vi "TrentVisionTest.vi"() -> ()   [LabVIEW 2011]
uses:
  <vilib>/Analysis/1siggen.llb/Ramp Pattern by Samples.vi
  <vilib>/Analysis/NI_AALBase.lvlib
  <vilib>/robotics/Navigation/shared/WorldMap/OccupancyGridWorldMap/NI_Robotics_OccupancyGridWorldMap.lvclass
panel:
  out "Image Out 2":T1(plugin-control)
  out "Lines Calibrated (Shape Detection 1) 2":T2(array[cluster]) {"End Point"."Y" format="%.2f"; "End Point"."X" format="%.2f"; "Start Point"."Y" format="%.2f"; "Start Point"."X" format="%.2f"}
  in  "ALL STOP":bool
  out "Started Scanning":bool
  in  "Step Over":bool
  out "Elapsed Time to Scan for First Time (sec)":dbl
  in  "Step Enable":bool
  out "Occupancy Grid":dbl[][](graph)
  out "XY Graph":cluster{dbl[], dbl[]}[](graph)
  in  "x Offset":i32
  in  "y Offset":i32
  in  "end point (135°)":dbl=100.0
  in  "Resulotion Controller\n1m = 10 units\n30m = 300 units (default)":i32=300
  in  "y start":i32
  in  "x start":i32
  out "Lines Calibrated (Shape Detection 1)":T2(array[cluster]) {"End Point"."Y" format="%.2f"; "End Point"."X" format="%.2f"; "Start Point"."Y" format="%.2f"; "Start Point"."X" format="%.2f"}
  out "Image Out":T1(plugin-control)
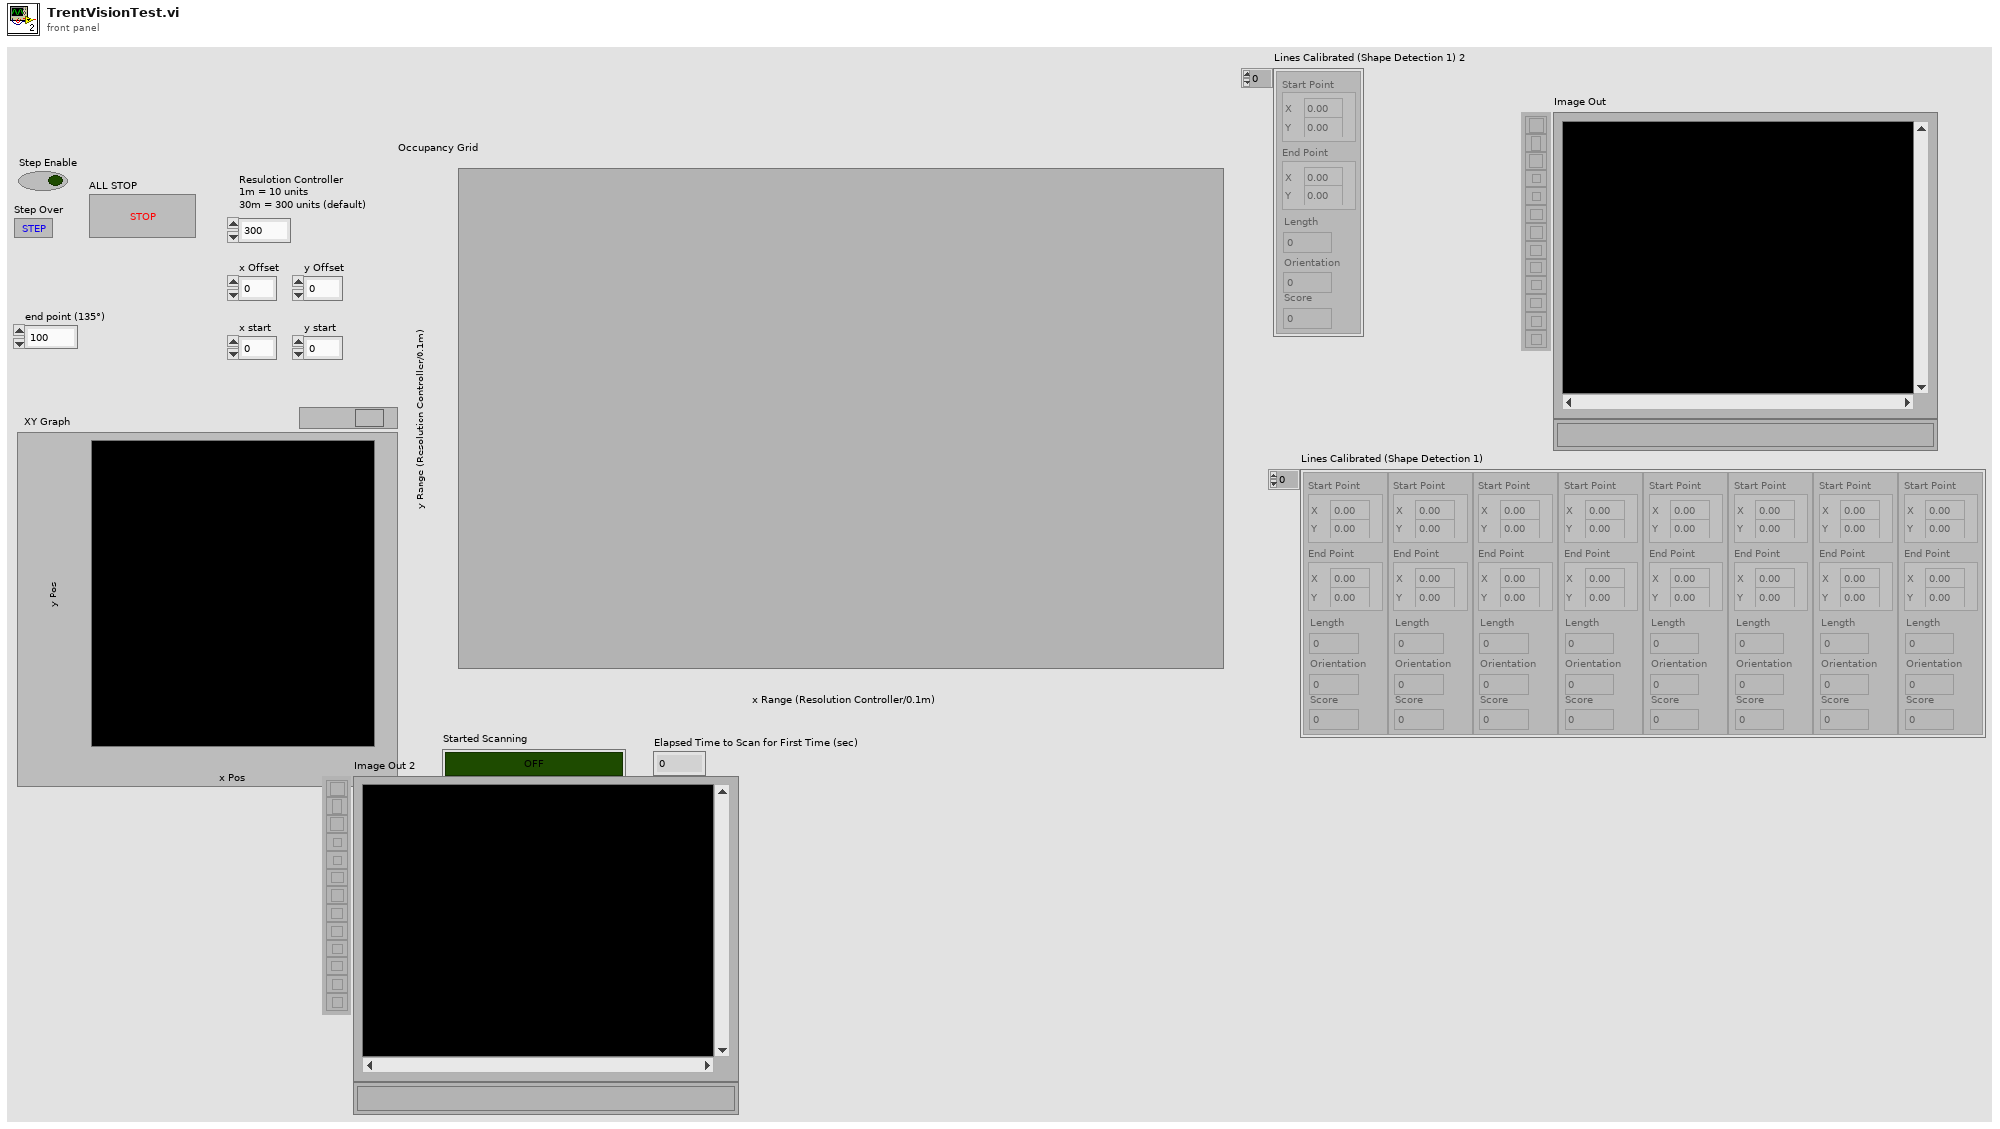
[diagram p1: front panel]
types:
  T1 = typedef "IMAQ Image.ctl" = refnum<image>
  T2 = cluster{"Start Point":cluster{"X":sgl, "Y":sgl}, "End Point":cluster{"X":sgl, "Y":sgl}, "Length":dbl, "Orientation":dbl, "Score":dbl}[]
  T3 = typedef "Image Type" = u32
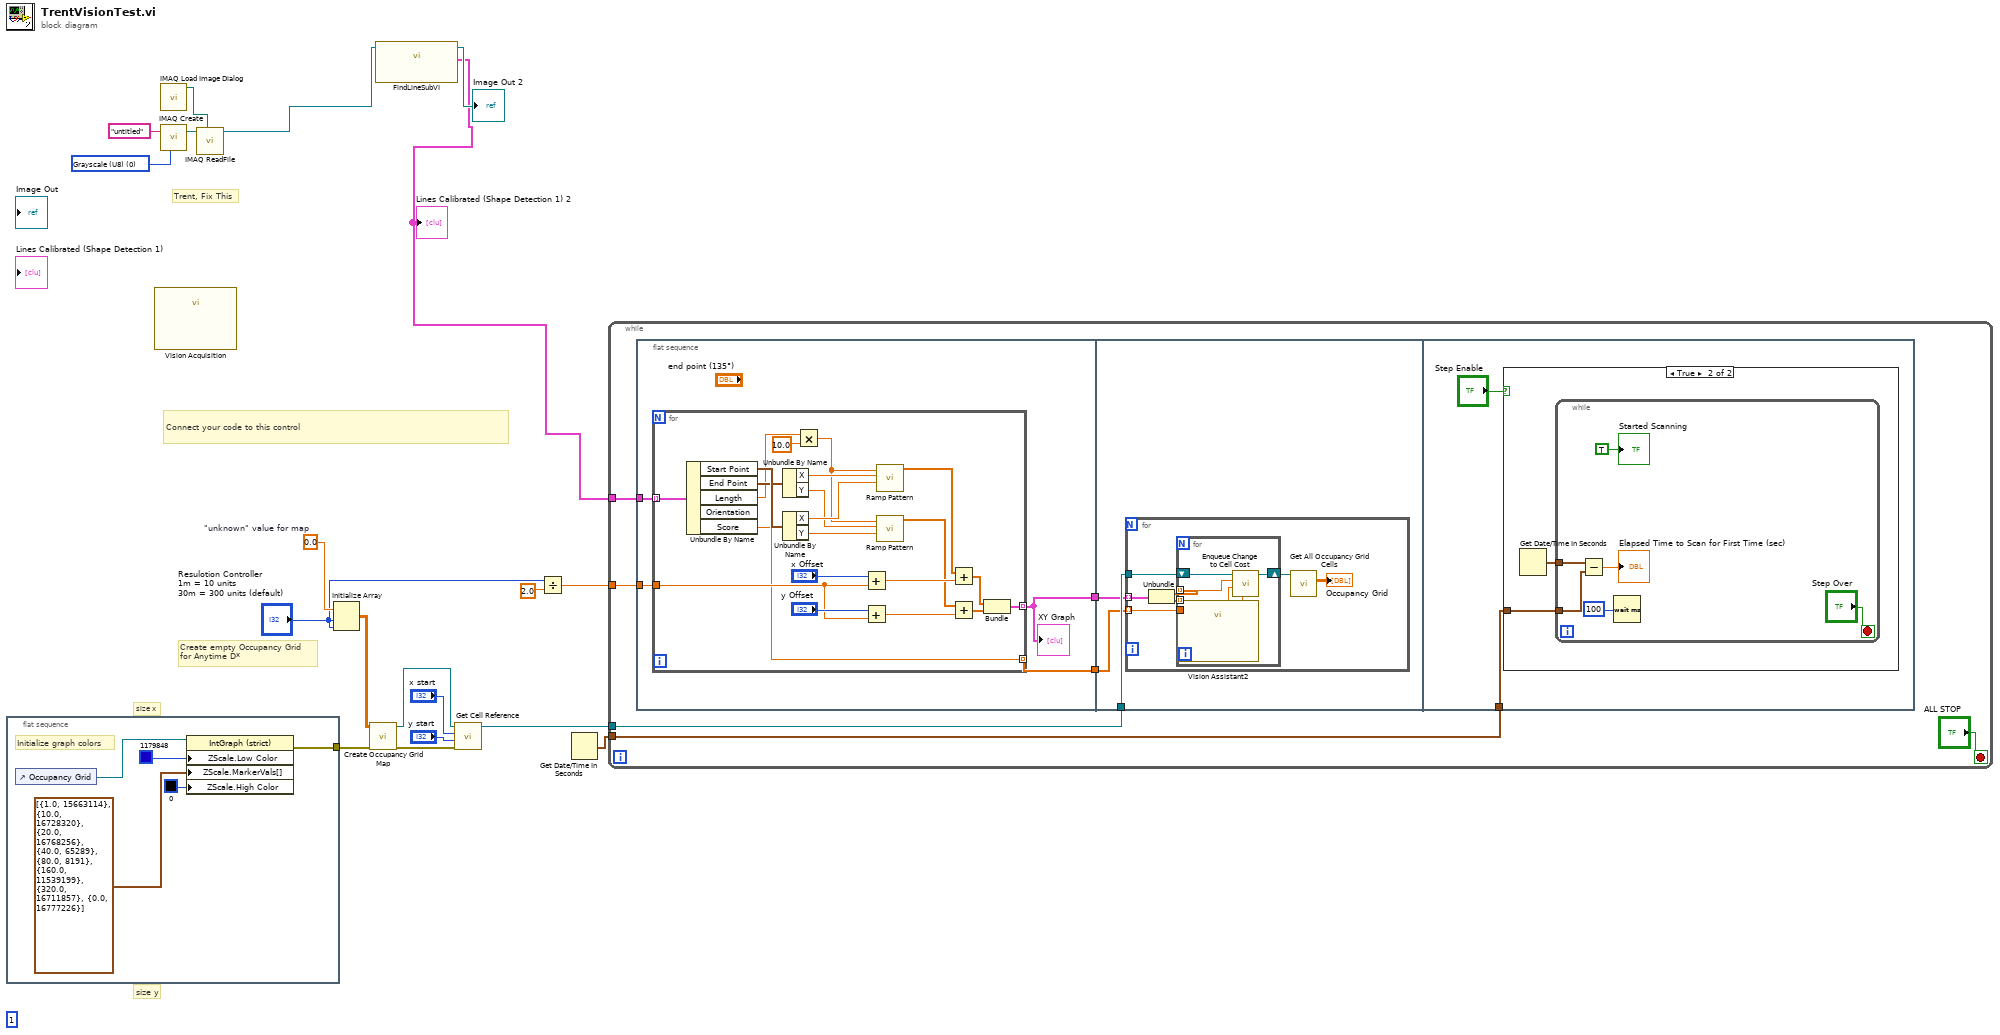
[diagram p0: block diagram]
diagram:
  w4 = T3 0 items=["Grayscale (U8)", "Grayscale (I16)", "Grayscale (SGL)", "Complex (CSG)", "RGB (U32)", "HSL (U32)", "RGB (U64)", "Grayscale (U16)"] ("Image Type")
  (unwired) 1
  w19 = 0.0  # "unknown" value for map
  # "Trent, Fix This"
  # "Connect your code to this control"
  # "size y"
  # "size x"
  # "Create empty Occupancy Grid\nfor Anytime D*"
  n1 = flat-sequence {
    tunnel: [w21] -> w13
    frame #0 {
      # "Initialize graph colors"
      n2 = control-ref of="Occupancy Grid"() -> (w20:refnum<vi>)
      n3 = property on="Property Node" class="IntGraph (strict)"(reference=w20, "ZScale.Low Color"=u32 1179848, "ZScale.MarkerVals[]"=cluster{dbl, u32}[] [{1.0, 15663114}, {10.0, 16728320}, {20.0, 16768256}, {40.0, 65289}, {80.0, 8191}, {160.0, 11539199}, {320.0, 16711857}, {0.0, 16777226}], "ZScale.High Color"=u32 0) -> (error out=w21:errorcluster)  [unwired: 1 in, 1 out]
    }
  }
  n4 = call "Vision Acquisition"() -> ()  [unwired: 20 in]
  n5 = call "IMAQ Load Image Dialog"() -> ("Path"=w5:path)  [unwired: 9 in, 2 out]
  n6 = call "IMAQ Create"("Image Name"="untitled", "Image Type"=w4) -> ("New Image"=w7:T1)  [unwired: 3 in, 1 out]
  n7 = call "IMAQ ReadFile"("File Path"=w5, "Image"=w7) -> ("Image Out"=w3:T1)  [unwired: 5 in, 4 out]
  n8 = Initialize Array(w19, "Resulotion Controller\n1m = 10 units\n30m = 300 units (default)", "Resulotion Controller\n1m = 10 units\n30m = 300 units (default)") -> (w18:dbl[][])
  n9 = call <vilib>:"Create Occupancy Grid Map.vi"("error in (no error)"=w13, "occupancy grid"=w18) -> ("error out"=w17:errorcluster, "map reference out"=w14:refnum<data-value>)  [unwired: 8 in]
  n10 = call "FindLineSubVI.vi"("Image In"=w3) -> ("Image Out"=→"Image Out 2":T1, "Lines Calibrated (Shape Detection 1)"=w1:T2)  [unwired: 24 in, 1 out]
  "Lines Calibrated (Shape Detection 1) 2" <- w1
  n11 = call <vilib>:"Get Cell Reference.vi"("error in (no error)"=w17, "y"="y start", "x"="x start", "map reference in"=w14) -> ("map reference out"=w12:refnum<data-value>)  [unwired: 4 in, 3 out]
  n12 = Divide(x="Resulotion Controller\n1m = 10 units\n30m = 300 units (default)", y=2.0) -> (x/y=w9:dbl)
  n13 = Get Date/Time In Seconds() -> (seconds since 1Jan1904=w8:timestamp)
  n14 = while {
    tunnel: w12 -> [w31]
    tunnel: w9 -> [w29]
    tunnel: w8 -> [w30]
    tunnel: w1 -> [w27]
    stop <- "ALL STOP" stop-if-true
    n15 = flat-sequence {
      tunnel: w29 -> [w35]
      tunnel: w27 -> [w34]
      tunnel: [w33] -> w26
      tunnel: [w32] -> w25
      tunnel: w31 -> [w59]
      tunnel: w26 -> [w58]
      tunnel: w25 -> [w57]
      tunnel: w30 -> [w73]
      frame #0 {
        n16 = for {
          tunnel: w34 -> [w56] mode=indexing
          tunnel: [w39] -> w33 mode=indexing
          tunnel: w35 -> [w37]
          tunnel: [w36] -> w32 mode=indexing
          n17 = Unbundle By Name(w56) -> ("Start Point"=w55:cluster{"X":sgl, "Y":sgl}, "End Point"=w54:cluster{"X":sgl, "Y":sgl}, "Length"=w48:dbl, "Score"=w36:dbl)  [unwired: 1 out]
          n18 = Unbundle By Name(w54) -> ("X"=w52:sgl, "Y"=w51:sgl)
          n19 = Unbundle By Name(w55) -> ("X"=w53:sgl, "Y"=w50:sgl)
          n20 = Multiply(x=w48, y=10.0) -> (x*y=w47:dbl)
          n21 = Add(x="x Offset", y=w37) -> (x+y=w44:dbl)
          n22 = Add(x="y Offset", y=w37) -> (x+y=w45:dbl)
          n23 = call-poly <vilib>:"Ramp Pattern.vi"("start"=w53, "end"=w52, "samples"=w47) -> ("Ramp Pattern"=w41:dbl[])  [unwired: 7 in, 1 out]
          n24 = call-poly <vilib>:"Ramp Pattern.vi"("start"=w50, "end"=w51, "samples"=w47) -> ("Ramp Pattern"=w40:dbl[])  [unwired: 7 in, 1 out]
          n25 = Add(x=w41, y=w44) -> (x+y=w42:dbl[])
          n26 = Add(x=w40, y=w45) -> (x+y=w43:dbl[])
          n27 = Bundle(w42, w43) -> (w39:cluster{dbl[], dbl[]})  [unwired: 1 out]
        }
        "XY Graph" <- w33
      }
      frame #1 {
        n28 = for {
          tunnel: w59 -> [w62]
          tunnel: w58 -> [w61] mode=indexing
          tunnel: w57 -> [w60] mode=indexing
          n29 = Unbundle(w61) -> (w63:dbl[], w64:dbl[])
          n30 = for {
            tunnel: w63 -> [w70] mode=indexing
            tunnel: w64 -> [w71] mode=indexing
            shift-right: [w68] -> w65
            shift-left: w62 -> [w69]
            tunnel: w60 -> [w67]
            n31 = call "Vision Assistant2"() -> ()  [unwired: 12 in]
            n32 = call <vilib>:"Enqueue Change to Cell Cost.vi"("cost"=w67, "y"=w71, "x"=w70, "map reference in"=w69) -> ("map reference out"=w68:refnum<data-value>)  [unwired: 6 in, 1 out]
          }
          n33 = call <vilib>:"Get All Occupancy Grid Cells.vi"("map reference in"=w65) -> ("occupancy grid"=→"Occupancy Grid":dbl[][])  [unwired: 8 in, 2 out]
        }
      }
      frame #2 {
        n34 = case shown="True" "Step Enable" {
          tunnel: w73 -> [_ w75]
          frame False {
          }
          frame True {
            n35 = Get Date/Time In Seconds() -> (seconds since 1Jan1904=w74:timestamp)
            n36 = while {
              tunnel: w75 -> [w78]
              tunnel: w74 -> [w76]
              stop <- "Step Over" stop-if-true
              n37 = Subtract(x=w76, y=w78) -> (x-y=→"Elapsed Time to Scan for First Time (sec)":dbl)
              n38 = Wait (ms)(milliseconds to wait=u32 100) -> ()  [unwired: 1 out]
              "Started Scanning" <- TRUE ("Boolean")
            }
          }
        }
      }
    }
  }
